vi "MercuryConfigured.vi"() -> ()   [LabVIEW 2013]
panel:
  out "Mercury Configured?":bool
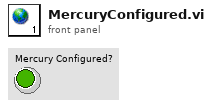
[diagram p1: front panel]
diagram:
